vi "BLM_ManualControl.vi"() -> ()   [LabVIEW 2018]
doc: "To start rotations:\n\nSelect The Motor (BLM) address\nRun this VI\nClick Test connection button\nClick INITIALIZE button \n (It is assumed that a BLM controller should be initialized only once: immediately after it is turned on. \n E.g., usually there is no need to initialize if you rebooted computer, but kept the motor controller on,\n the motor was connected to the controller and you wish to continue using current position counting. \n Initialization occurs only if the current motor position is equal to zero.) \nClick READ BLM position button\nSelect desired MODE, SPEED, and Distance (or Final Position, depends on the MODE) value\nClick RUN BLM button\n\nSET POSITION button does not affect actual sample/motor position, but changes the position value\nin the controller memory. Thus, it allows to assign any value to the current motor position.\n\nSee also:\nhttps://opswiki.magnet.fsu.edu/wiki/pages/K7Q8u4C4s9/Rotating_probes_equipped_with_Brushless_Motors_BLMs.html\n\nNHMFL; A.Suslov; Feb 2012; updated Aug 2016"
uses:
  IMS Stepper Controller/stepper motor action.ctl
  slider setter action.ctl
panel:
  out "Error Out":errorcluster {"code" format="%.0x"}
  in  "MODE:":enum32{"ABSOLUTE", "INCREMENTAL"}(radio)=enum."INCREMENTAL"
  in  "Read Position":bool
  out "Test Results":string
  in  "Test Connection":bool
  out "BLM Position":dbl caption="BLM position\nincrement 0.045 \n (deg of BLM)" format="%.3f"
  in  "Parameter changed":bool
  in  "stop":bool
  in  "Set Position":bool
  in  "INITIALIZE":bool
  in  "Run":bool
  in  "New position":dbl caption="Final position:\nincrement 0.045 \n (deg of BLM)" step=0.045 format="%#.3g"
  in  "SPEED (rot/sec)\nincrement .0042":dbl=0.0294 min=0.0042 max=0.42 step=0.0042
  in  "MOTOR (BLM) Address":refnum<visa-resource-name>
  # "Select The Motor (BLM) address\nRun this VI\nClick Test connection button\nClick  INITIALIZE button \nClick  READ BLM position button\nSelect desired MODE, SPEED, and\n         Distance (or Final Position)\nClick RUN BLM button\n\nMore Help at File-> VI Propeties->\nDocumentation\nand Operations Wiki"
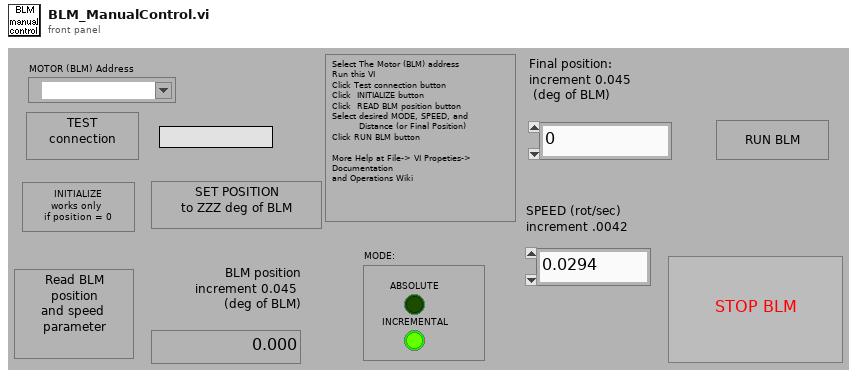
[diagram p1: front panel]
types:
  T1 = typedef "stepper motor action.ctl" = enum16{"go", "stop", "check", "init", "sync", "set", "set speed", "void"}
  T2 = enum8{"Enabled", "Disabled", "Disabled and Grayed Out"}
  T3 = typedef "slider setter action.ctl" = enum16{"--update circle", "set step slider moves", "cursor moves", "current pos changed", "init", "void", "--draw current lie", "--draw set line", "--move current step slider", "--move set step slider", "--draw limit lines", "check", "--move set angle slider", "--move current angle slider", "set angle slider moves", "--move cursor", "set set step", "set current step"}
  T4 = typedef "stepper motor state.ctl" = enum16{"moving", "stopped"}
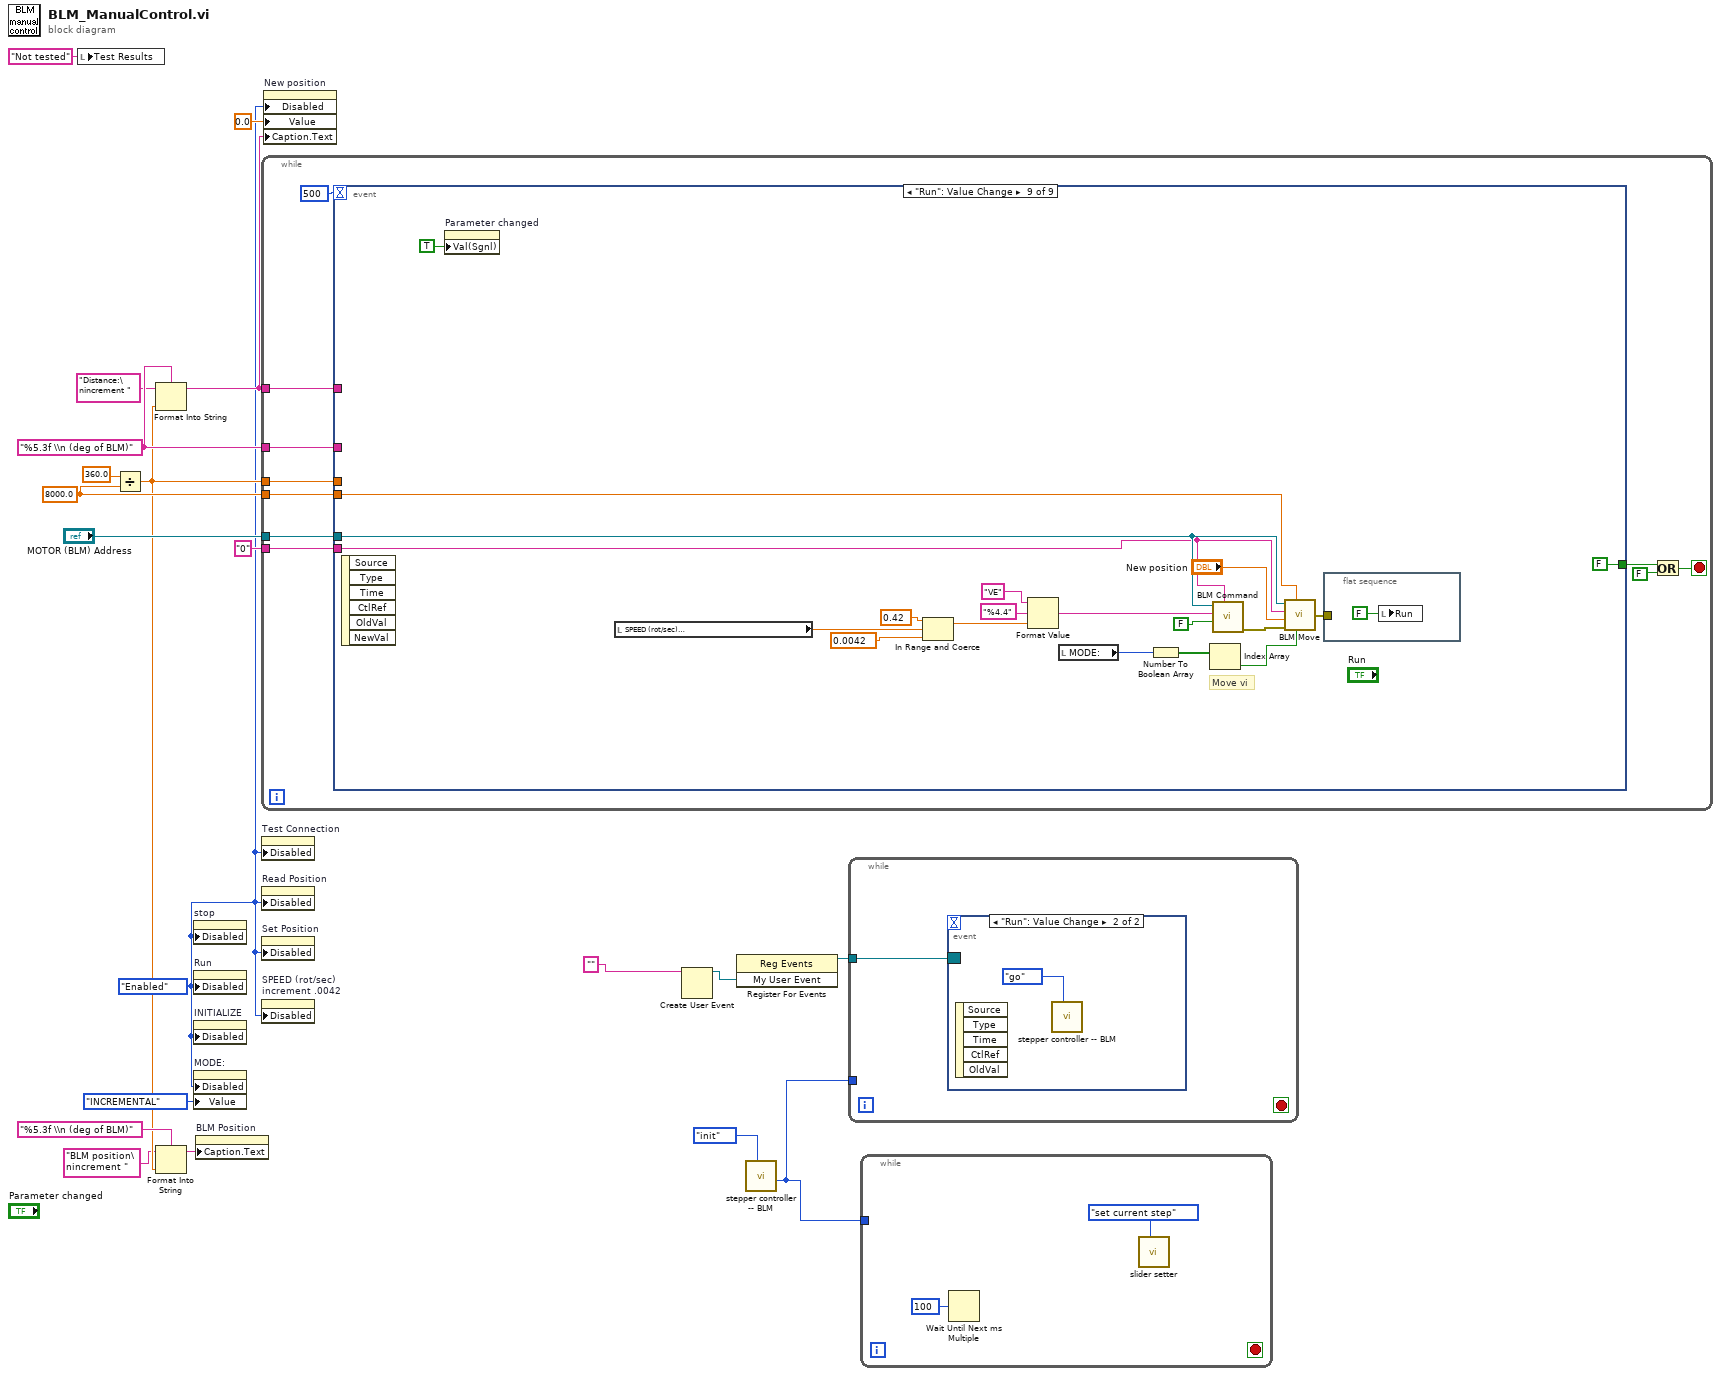
[diagram p0: block diagram]
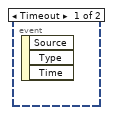
[diagram p2: hidden frame]
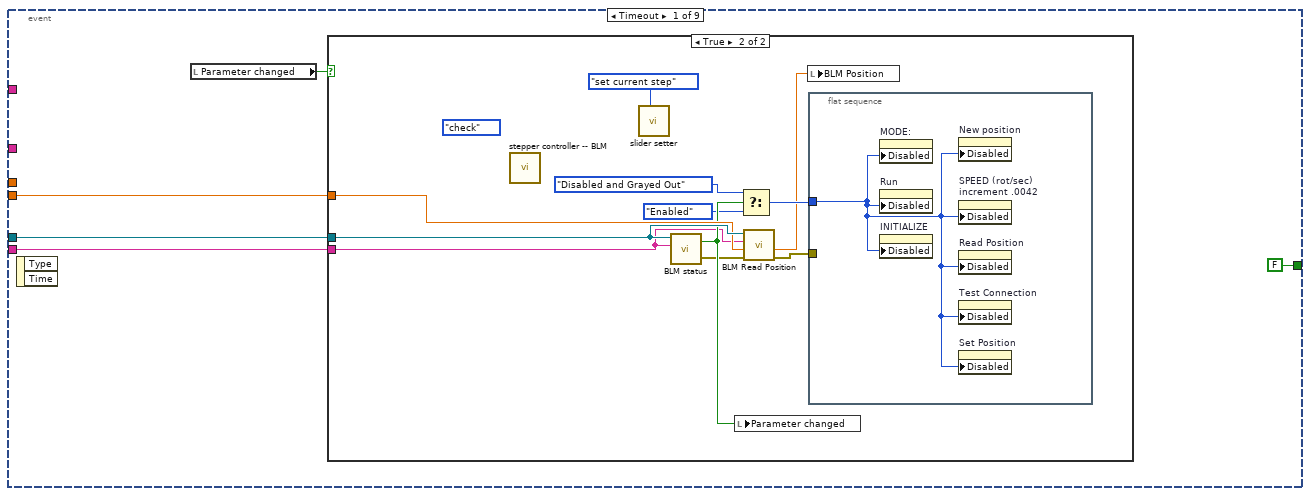
[diagram p3: hidden frame]
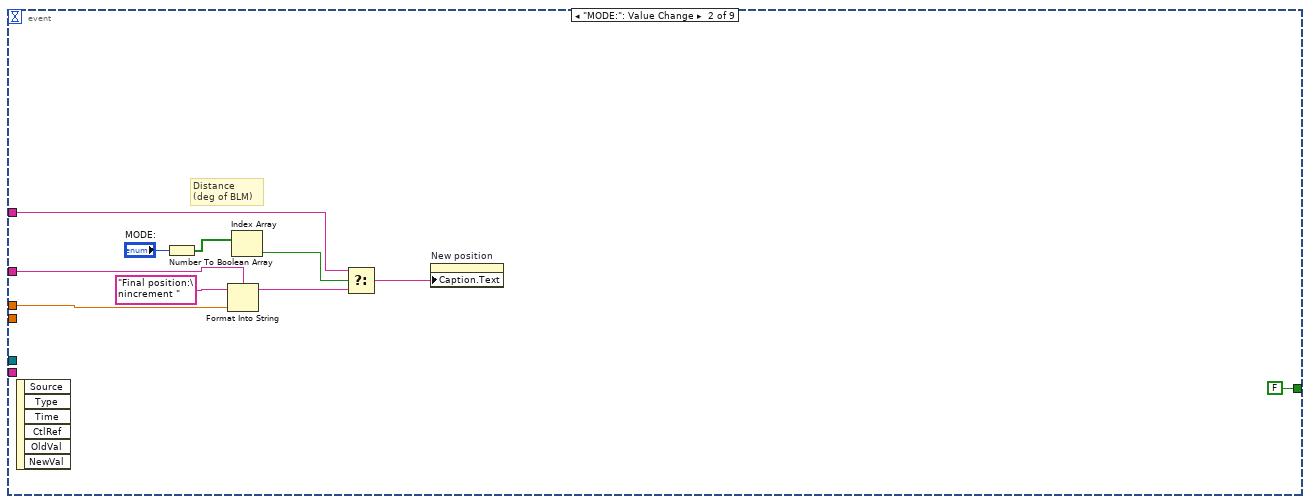
[diagram p5: hidden frame]
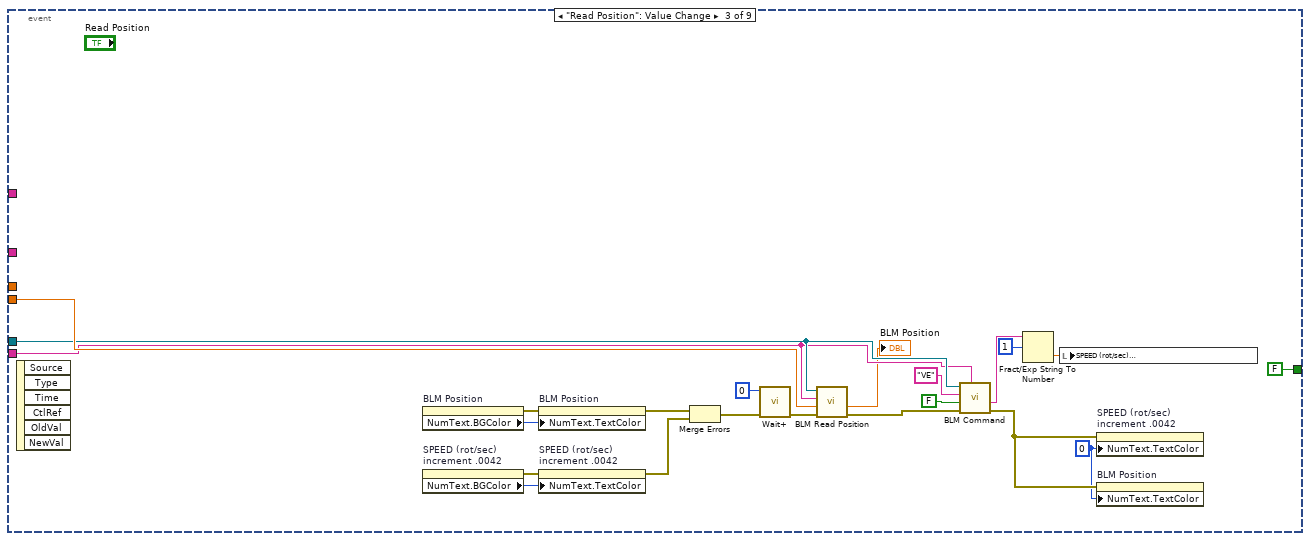
[diagram p6: hidden frame]
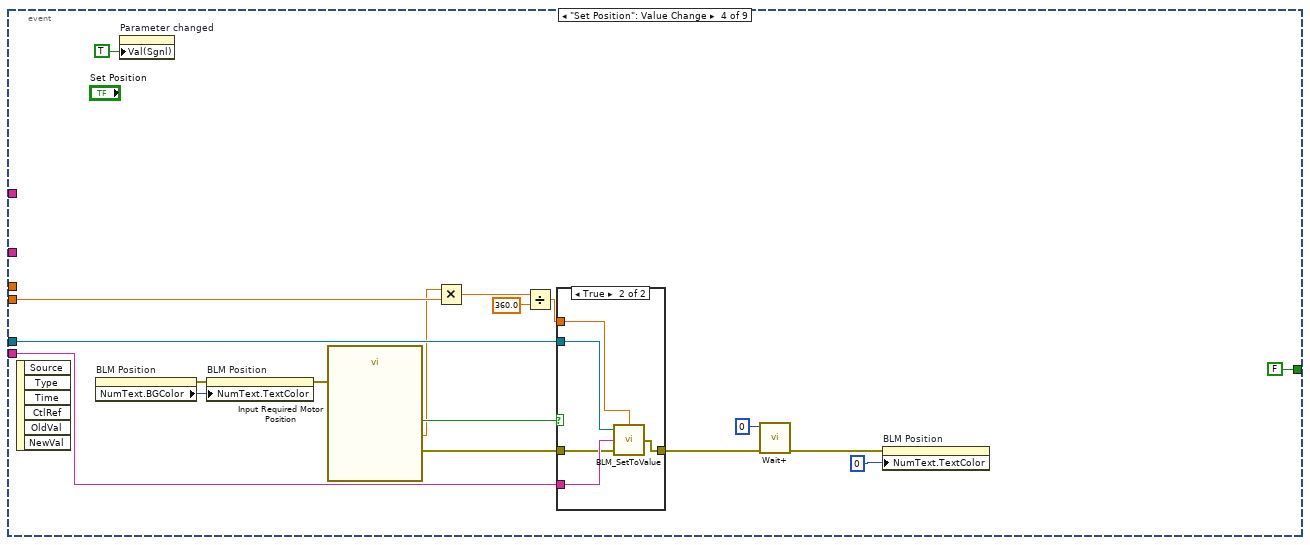
[diagram p7: hidden frame]
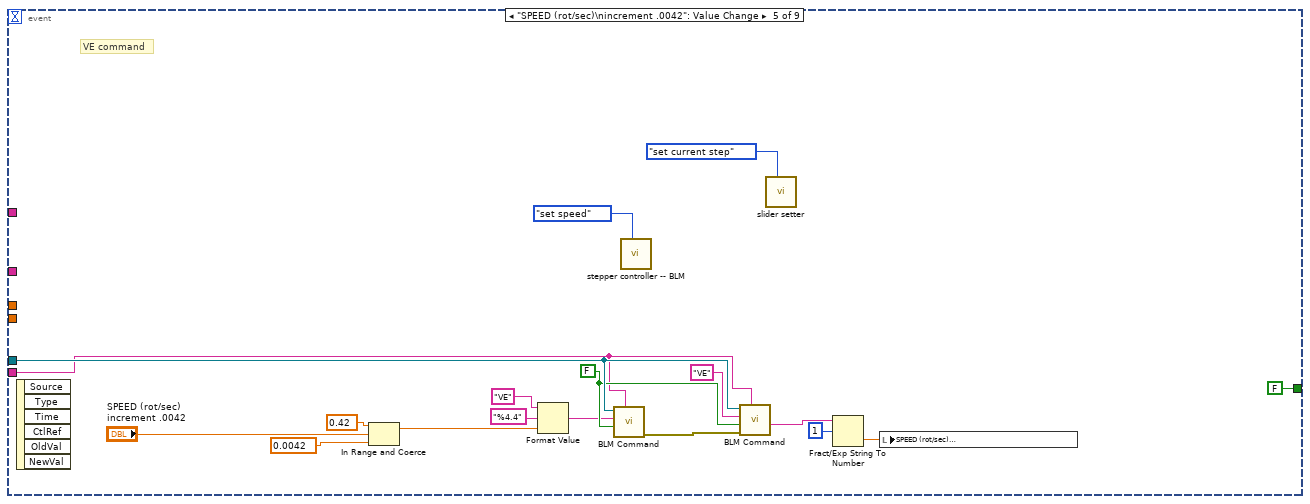
[diagram p9: hidden frame]
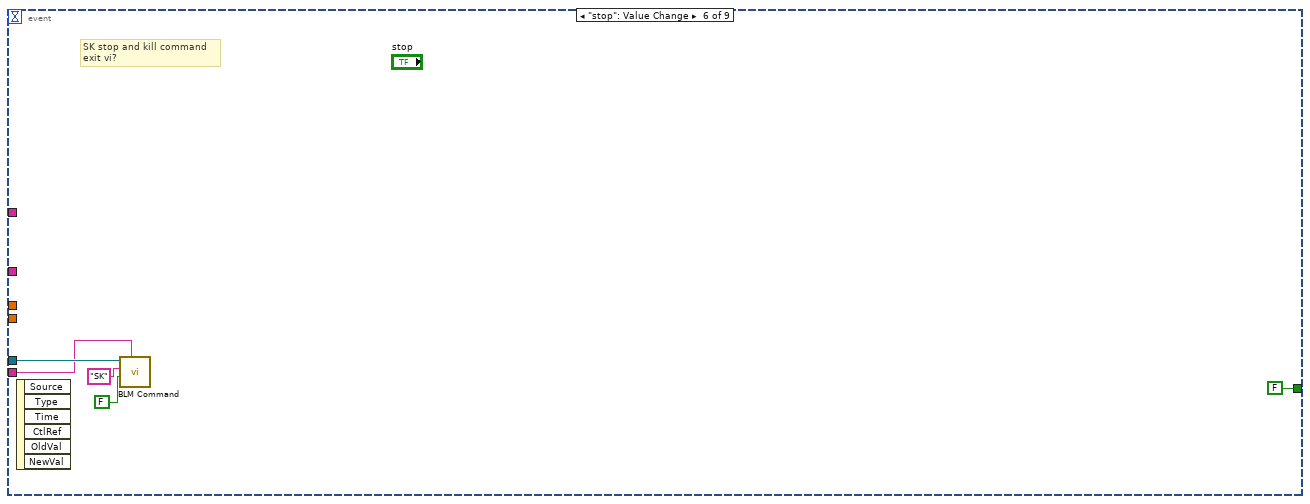
[diagram p10: hidden frame]
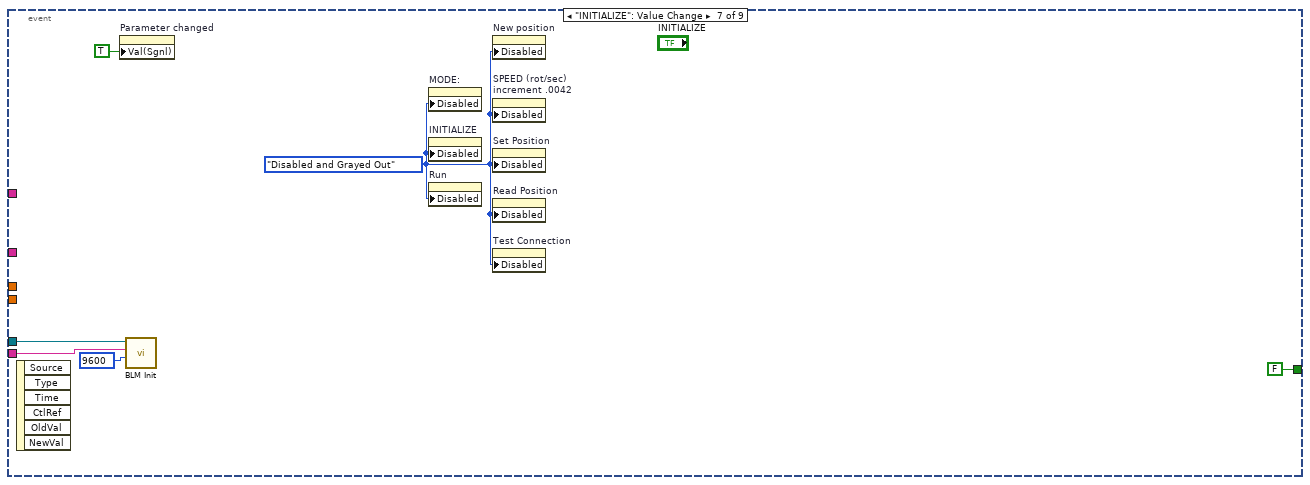
[diagram p11: hidden frame]
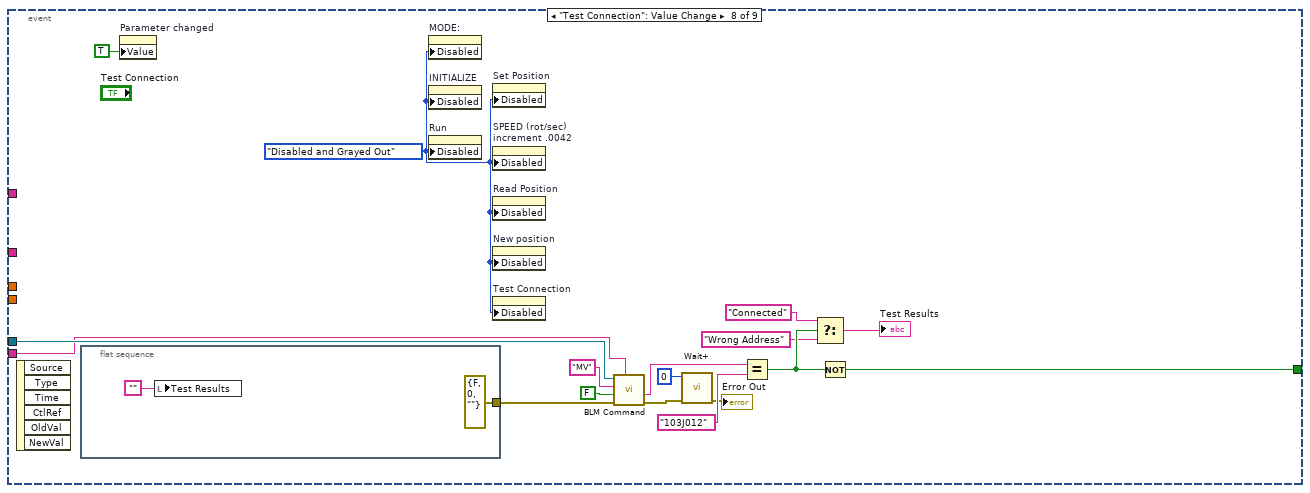
[diagram p12: hidden frame]
diagram:
  w7 = T2."Enabled" ("Disabled")
  w13 = "%5.3f \\n (deg of BLM)" ("format string")
  w15 = 8000.0 ("Steps/rot")
  n1 = local write "Test Results"("Not tested" ("s? t:f")) -> ()
  n2 = Divide(x=360.0, y=w15) -> (x/y=w10:dbl)
  n3 = Format Into String(format string=w13, initial string="Distance:\nincrement " ("Label.Text"), w10) -> (resulting string=w14:string)  [unwired: 1 in, 1 out]
  n4 = Format Into String(format string="%5.3f \\n (deg of BLM)", initial string="BLM position\nincrement ", w10) -> (resulting string=w11:string)  [unwired: 1 in, 1 out]
  n5 = property on="stop" class="Bool"("Disabled"=w7) -> ()  [unwired: 2 in, 2 out]
  n6 = property on="Run" class="Bool (strict)"("Disabled"=w7) -> ()  [unwired: 2 in, 2 out]
  n7 = property on="INITIALIZE" class="Bool"("Disabled"=w7) -> ()  [unwired: 2 in, 2 out]
  n8 = property on="MODE:" class="RadioBtnsControl (strict)"("Disabled"=w7, "Value"=enum32{"ABSOLUTE", "INCREMENTAL"}."INCREMENTAL" ("MODE:")) -> ()  [unwired: 2 in, 2 out]
  n9 = property on="BLM Position" class="DigNum (strict)"("Caption.Text"=w11) -> ()  [unwired: 2 in, 2 out]
  n10 = while {
    tunnel: w15 -> [w30]
    tunnel: "MOTOR (BLM) Address" -> [w29]
    tunnel: w14 -> [w24]
    tunnel: "0" ("Motor Address") -> [w23]
    tunnel: w10 -> [w22]
    tunnel: w13 -> [w21]
    stop <- w26 stop-if-true
    n11 = event shown="[8] \"Run\": Value Change" {
      selector: _ -> [_ _ _ _ _ _ _ _ _]
      dyn-events: _ -> [_ _ _ _ _ _ _ _ _]
      timeout: 500 -> [_ _ _ _ _ _ _ _ _]
      tunnel: w30 -> [w34 _ w79 w94 _ _ _ _ w170]
      tunnel: w29 -> [w35 _ w78 w97 w121 w126 w131 w149 w169]
      tunnel: [FALSE FALSE FALSE FALSE FALSE FALSE FALSE w147 FALSE] -> w25
      tunnel: w24 -> [_ w56 _ _ _ _ _ _ _]
      tunnel: w23 -> [w32 _ w77 w95 w117 w123 w129 w145 w167]
      tunnel: w22 -> [_ w50 _ _ _ _ _ _ _]
      tunnel: w21 -> [_ w49 _ _ _ _ _ _ _]
      event Timeout {
        n12 = event-data() -> ()  [unwired: 1 in, 2 out]
        n13 = local read "Parameter changed"() -> (w33:bool)
        n14 = case shown="True" w33 {
          tunnel: w35 -> [_ w46]
          tunnel: w34 -> [_ w45]
          tunnel: w32 -> [_ w41]
          frame False {
          }
          frame True {
            (unwired) stepper_motor_action."check" ("stepper motor action")
            n15 = call "stepper controller -- BLM.vi"() -> ()  [unwired: 11 in, 1 out]
            n16 = call "slider setter.vi"("slider setter action"=slider_setter_action."set current step") -> ()  [unwired: 10 in, 1 out]
            n17 = call "BLM status.vi"("Motor Address"=w41, "Porty Address"=w46) -> ("error out"=w40:errorcluster, "Motor is moving"=w44:bool)  [unwired: 2 in]
            n18 = local write "Parameter changed"(w44) -> ()
            n19 = Select(t=T2."Disabled and Grayed Out" ("Disabled"), s=w44, f=T2."Enabled" ("Disabled")) -> (s? t:f=w43:T2)
            n20 = call "BLM Read Position.vi"("error in (no error)"=w40, "Steps/rot"=w45, "Motor Address"=w41, "Port Address"=w46) -> ("error out"=w39:errorcluster, "Response"=w42:dbl)  [unwired: 2 out]
            n21 = local write "BLM Position"(w42) -> ()
            n22 = flat-sequence {
              tunnel: w43 -> [w47]
              tunnel: w39 -> [_]
              frame #0 {
                n23 = property on="MODE:" class="RadioBtnsControl (strict)"("Disabled"=w47) -> ()  [unwired: 2 in, 2 out]
                n24 = property on="Run" class="Bool (strict)"("Disabled"=w47) -> ()  [unwired: 2 in, 2 out]
                n25 = property on="INITIALIZE" class="Bool"("Disabled"=w47) -> ()  [unwired: 2 in, 2 out]
                n26 = property on="New position" class="DigNum (strict)"("Disabled"=w47) -> ()  [unwired: 2 in, 2 out]
                n27 = property on="SPEED (rot/sec)\nincrement .0042" class="DigNum (strict)"("Disabled"=w47) -> ()  [unwired: 2 in, 2 out]
                n28 = property on="Read Position" class="Bool"("Disabled"=w47) -> ()  [unwired: 2 in, 2 out]
                n29 = property on="Test Connection" class="Bool"("Disabled"=w47) -> ()  [unwired: 2 in, 2 out]
                n30 = property on="Set Position" class="Bool"("Disabled"=w47) -> ()  [unwired: 2 in, 2 out]
              }
            }
          }
        }
      }
      event "MODE:": Value Change {
        # "Distance  \n(deg of BLM)"
        n31 = event-data() -> ()  [unwired: 1 in, 6 out]
        n32 = Number To Boolean Array(number="MODE:") -> (Boolean array=w54:bool[])
        n33 = Format Into String(format string=w49, initial string="Final position:\nincrement " ("f"), w50) -> (resulting string=w52:string)  [unwired: 1 in, 1 out]
        n34 = Index Array(array=w54) -> (element=w53:bool)  [unwired: 1 in]
        n35 = Select(t=w56, s=w53, f=w52) -> (s? t:f=w57:string)
        n36 = property on="New position" class="DigNum (strict)"("Caption.Text"=w57) -> ()  [unwired: 2 in, 2 out]
      }
      event "Read Position": Value Change {
        w64 = u32 0 ("Numeric Text.Text Colors:Text Color")
        n37 = event-data() -> ()  [unwired: 1 in, 6 out]
        n38 = property on="BLM Position" class="DigNum (strict)"() -> (error out=w58:errorcluster, "NumText.BGColor"=w63:u32)  [unwired: 2 in, 1 out]
        n39 = property on="SPEED (rot/sec)\nincrement .0042" class="DigNum (strict)"() -> (error out=w59:errorcluster, "NumText.BGColor"=w62:u32)  [unwired: 2 in, 1 out]
        n40 = property on="BLM Position" class="DigNum (strict)"(error in=w58, "NumText.TextColor"=w63) -> (error out=w61:errorcluster)  [unwired: 1 in, 1 out]
        n41 = property on="SPEED (rot/sec)\nincrement .0042" class="DigNum (strict)"(error in=w59, "NumText.TextColor"=w62) -> (error out=w60:errorcluster)  [unwired: 1 in, 1 out]
        n42 = Merge Errors(w61, w60) -> (w65:errorcluster)
        n43 = call "Wait+.vi"("Error In"=w65, "milliseconds to wait"=u32 0 ("millisecond timer value")) -> ("Error Out"=w67:errorcluster)  [unwired: 4 in, 1 out]
        n44 = call "BLM Read Position.vi"("error in (no error)"=w67, "Steps/rot"=w79, "Motor Address"=w77, "Port Address"=w78) -> ("error out"=w69:errorcluster, "Response"=→"BLM Position":dbl)  [unwired: 2 out]
        n45 = call "BLM Command.vi"("Motor Address"=w77, "error in (no error)"=w69, "Read Echo?"=FALSE, "Command"="VE", "Port Address"=w78) -> ("error out"=w75:errorcluster, "Response"=w72:string)  [unwired: 1 in, 3 out]
        n46 = Fract/Exp String To Number(string=w72, offset=1) -> (number=w70:dbl)  [unwired: 2 in, 1 out]
        n47 = local write "SPEED (rot/sec)\nincrement .0042"(w70) -> ()
        n48 = property on="SPEED (rot/sec)\nincrement .0042" class="DigNum (strict)"(error in=w75, "NumText.TextColor"=w64) -> ()  [unwired: 1 in, 2 out]
        n49 = property on="BLM Position" class="DigNum (strict)"(error in=w75, "NumText.TextColor"=w64) -> ()  [unwired: 1 in, 2 out]
      }
      event "Set Position": Value Change {
        n50 = event-data() -> ()  [unwired: 1 in, 6 out]
        n51 = property on="BLM Position" class="DigNum (strict)"() -> (error out=w80:errorcluster, "NumText.BGColor"=w89:u32)  [unwired: 2 in, 1 out]
        n52 = property on="Parameter changed" class="Bool (strict)"("Val(Sgnl)"=TRUE ("Value (Signaling)")) -> ()  [unwired: 2 in, 2 out]
        n53 = property on="BLM Position" class="DigNum (strict)"(error in=w80, "NumText.TextColor"=w89) -> (error out=w90:errorcluster)  [unwired: 1 in, 1 out]
        n54 = call "Input Required Motor Position"("error in (no error)"=w90) -> ("Position:"=w87:dbl, "OK"=w88:bool, "error out"=w83:errorcluster)  [unwired: 16 in]
        n55 = Multiply(x=w87, y=w94) -> (x*y=w85:dbl)
        n56 = Divide(x=w85, y=360.0) -> (x/y=w86:dbl)
        n57 = case shown="True" w88 {
          tunnel: w97 -> [_ w103]
          tunnel: w95 -> [_ w102]
          tunnel: w86 -> [_ w101]
          tunnel: [w98 w100] -> w92
          tunnel: w83 -> [w98 w99]
          frame False {
          }
          frame True {
            n58 = call "BLM_SetToValue.vi"("Position"=w101, "error in (no error)"=w99, "Motor Address"=w102, "Port Address"=w103) -> ("error out"=w100:errorcluster)
          }
        }
        n59 = call "Wait+.vi"("Error In"=w92, "milliseconds to wait"=u32 0) -> ("Error Out"=w91:errorcluster)  [unwired: 4 in, 1 out]
        n60 = property on="BLM Position" class="DigNum (strict)"(error in=w91, "NumText.TextColor"=u32 0 ("Numeric Text.Text Colors:Text Color")) -> ()  [unwired: 1 in, 2 out]
      }
      event "SPEED (rot/sec)\nincrement .0042": Value Change {
        w120 = FALSE
        # "VE command"
        n61 = event-data() -> ()  [unwired: 1 in, 6 out]
        n62 = In Range and Coerce(upper limit=0.42 ("x"), x="SPEED (rot/sec)\nincrement .0042", lower limit=0.0042) -> (coerced(x)=w113:dbl)  [unwired: 1 out]
        n63 = Format Value(string ("")="VE", format string="%4.4", value (0)=w113) -> (output string=w110:string)
        n64 = call "BLM Command.vi"("Motor Address"=w117, "Read Echo?"=w120, "Command"=w110, "Port Address"=w121) -> ("error out"=w118:errorcluster)  [unwired: 2 in, 4 out]
        n65 = call "stepper controller -- BLM.vi"("stepper driver action"=stepper_motor_action."set speed" ("stepper motor action")) -> ()  [unwired: 10 in, 1 out]
        n66 = call "BLM Command.vi"("Motor Address"=w117, "error in (no error)"=w118, "Read Echo?"=w120, "Command"="VE", "Port Address"=w121) -> ("Response"=w107:string)  [unwired: 1 in, 4 out]
        n67 = call "slider setter.vi"("slider setter action"=slider_setter_action."set current step") -> ()  [unwired: 10 in, 1 out]
        n68 = Fract/Exp String To Number(string=w107, offset=1) -> (number=w119:dbl)  [unwired: 2 in, 1 out]
        n69 = local write "SPEED (rot/sec)\nincrement .0042"(w119) -> ()
      }
      event "stop": Value Change {
        # "SK stop and kill command\nexit vi?"
        n70 = event-data() -> ()  [unwired: 1 in, 6 out]
        n71 = call "BLM Command.vi"("Motor Address"=w123, "Read Echo?"=FALSE, "Command"="SK", "Port Address"=w126) -> ()  [unwired: 2 in, 5 out]
      }
      event "INITIALIZE": Value Change {
        w127 = T2."Disabled and Grayed Out" ("Disabled")
        n72 = event-data() -> ()  [unwired: 1 in, 6 out]
        n73 = property on="Parameter changed" class="Bool (strict)"("Val(Sgnl)"=TRUE ("Value (Signaling)")) -> ()  [unwired: 2 in, 2 out]
        n74 = call "BLM Init.vi"("Baud Rate"=u32 9600, "Motor Address"=w129, "Port Address"=w131) -> ()  [unwired: 1 in, 3 out]
        n75 = property on="MODE:" class="RadioBtnsControl (strict)"("Disabled"=w127) -> ()  [unwired: 2 in, 2 out]
        n76 = property on="INITIALIZE" class="Bool"("Disabled"=w127) -> ()  [unwired: 2 in, 2 out]
        n77 = property on="Run" class="Bool (strict)"("Disabled"=w127) -> ()  [unwired: 2 in, 2 out]
        n78 = property on="New position" class="DigNum (strict)"("Disabled"=w127) -> ()  [unwired: 2 in, 2 out]
        n79 = property on="SPEED (rot/sec)\nincrement .0042" class="DigNum (strict)"("Disabled"=w127) -> ()  [unwired: 2 in, 2 out]
        n80 = property on="Set Position" class="Bool"("Disabled"=w127) -> ()  [unwired: 2 in, 2 out]
        n81 = property on="Read Position" class="Bool"("Disabled"=w127) -> ()  [unwired: 2 in, 2 out]
        n82 = property on="Test Connection" class="Bool"("Disabled"=w127) -> ()  [unwired: 2 in, 2 out]
      }
      event "Test Connection": Value Change {
        w144 = T2."Disabled and Grayed Out" ("Disabled")
        n83 = event-data() -> ()  [unwired: 1 in, 6 out]
        n84 = flat-sequence {
          tunnel: [errorcluster {"status"=FALSE, "code"=0, "source"=""} ("error in (no error)")] -> w134
          frame #0 {
            n85 = local write "Test Results"("" ("Response")) -> ()
          }
        }
        n86 = property on="Parameter changed" class="Bool (strict)"("Value"=TRUE ("Parameter changed")) -> ()  [unwired: 2 in, 2 out]
        n87 = property on="MODE:" class="RadioBtnsControl (strict)"("Disabled"=w144) -> ()  [unwired: 2 in, 2 out]
        n88 = property on="INITIALIZE" class="Bool"("Disabled"=w144) -> ()  [unwired: 2 in, 2 out]
        n89 = property on="Run" class="Bool (strict)"("Disabled"=w144) -> ()  [unwired: 2 in, 2 out]
        n90 = property on="Set Position" class="Bool"("Disabled"=w144) -> ()  [unwired: 2 in, 2 out]
        n91 = property on="SPEED (rot/sec)\nincrement .0042" class="DigNum (strict)"("Disabled"=w144) -> ()  [unwired: 2 in, 2 out]
        n92 = property on="Read Position" class="Bool"("Disabled"=w144) -> ()  [unwired: 2 in, 2 out]
        n93 = property on="New position" class="DigNum (strict)"("Disabled"=w144) -> ()  [unwired: 2 in, 2 out]
        n94 = property on="Test Connection" class="Bool"("Disabled"=w144) -> ()  [unwired: 2 in, 2 out]
        n95 = call "BLM Command.vi"("Motor Address"=w145, "error in (no error)"=w134, "Read Echo?"=FALSE, "Command"="MV", "Port Address"=w149) -> ("error out"=w143:errorcluster, "Response"=w140:string)  [unwired: 1 in, 3 out]
        n96 = call "Wait+.vi"("Error In"=w143, "milliseconds to wait"=u32 0) -> ("Error Out"=→"Error Out":errorcluster)  [unwired: 4 in, 1 out]
        n97 = Equal?(x=w140, y="103J012" ("Response")) -> (x = y?=w148:bool)
        n98 = Select(t="Connected" ("Response"), s=w148, f="Wrong Address" ("Response")) -> (s? t:f=→"Test Results":string)
        n99 = Not(x=w148) -> (.not. x?=w147:bool)
      }
      event "Run": Value Change {
        # "Move vi"
        n100 = event-data() -> ()  [unwired: 1 in, 6 out]
        n101 = property on="Parameter changed" class="Bool (strict)"("Val(Sgnl)"=TRUE ("Value (Signaling)")) -> ()  [unwired: 2 in, 2 out]
        n102 = local read "SPEED (rot/sec)\nincrement .0042"() -> (w168:dbl)
        n103 = In Range and Coerce(upper limit=0.42 ("x"), x=w168, lower limit=0.0042) -> (coerced(x)=w162:dbl)  [unwired: 1 out]
        n104 = Format Value(string ("")="VE", format string="%4.4", value (0)=w162) -> (output string=w158:string)
        n105 = local read "MODE:"() -> (w154:enum32{"ABSOLUTE", "INCREMENTAL"})
        n106 = Number To Boolean Array(number=w154) -> (Boolean array=w155:bool[])
        n107 = Index Array(array=w155) -> (element=w153:bool)  [unwired: 1 in]
        n108 = call "BLM Command.vi"("Motor Address"=w167, "Read Echo?"=FALSE, "Command"=w158, "Port Address"=w169) -> ("error out"=w166:errorcluster)  [unwired: 2 in, 4 out]
        n109 = call "BLM Move.vi"("Mode IS:"=w153, "Steps/rot"=w170, "error in (no error)"=w166, "Position / Distance"="New position", "Motor Address"=w167, "Port Address"=w169) -> ("error out"=w165:errorcluster)
        n110 = flat-sequence {
          tunnel: w165 -> [_]
          frame #0 {
            n111 = local write "Run"(FALSE ("Run")) -> ()
          }
        }
      }
    }
    n112 = Or(x=w25, y=FALSE) -> (x .or. y?=w26:bool)
  }
  n113 = property on="Test Connection" class="Bool"("Disabled"=w7) -> ()  [unwired: 2 in, 2 out]
  n114 = property on="Read Position" class="Bool"("Disabled"=w7) -> ()  [unwired: 2 in, 2 out]
  n115 = property on="Set Position" class="Bool"("Disabled"=w7) -> ()  [unwired: 2 in, 2 out]
  n116 = property on="SPEED (rot/sec)\nincrement .0042" class="DigNum (strict)"("Disabled"=w7) -> ()  [unwired: 2 in, 2 out]
  n117 = property on="New position" class="DigNum (strict)"("Disabled"=w7, "Value"=0.0 ("New position / \n distance (deg of BLM)"), "Caption.Text"=w14) -> ()  [unwired: 2 in, 2 out]
  n118 = Create User Event(user event datatype="") -> (user event=w3:refnum<user-event>)  [unwired: 1 in, 1 out]
  n119 = register-events(w3) -> (reference out=w5:refnum<event-registration>)  [unwired: 2 in, 1 out]
  n120 = call "stepper controller -- BLM.vi"("stepper driver action"=stepper_motor_action."init" ("stepper motor action")) -> ("stepper motor state OUT"=w1:T4)  [unwired: 10 in]
  n121 = while {
    tunnel: w5 -> [w172]
    tunnel: w1 -> [_]
    stop <- _ stop-if-true
    n122 = event shown="[1] \"Run\": Value Change" {
      selector: w172 -> [_ _]
      dyn-events: _ -> [_ _]
      timeout: _ -> [_ _]
      event Timeout {
        n123 = event-data() -> ()  [unwired: 1 in, 3 out]
      }
      event "Run": Value Change {
        n124 = event-data() -> ()  [unwired: 1 in, 5 out]
        n125 = call "stepper controller -- BLM.vi"("stepper driver action"=stepper_motor_action."go" ("stepper motor action")) -> ()  [unwired: 10 in, 1 out]
      }
    }
  }
  n126 = while {
    tunnel: w1 -> [_]
    stop <- _ stop-if-true
    n127 = Wait Until Next ms Multiple(millisecond multiple=u32 100) -> ()  [unwired: 1 out]
    n128 = call "slider setter.vi"("slider setter action"=slider_setter_action."set current step") -> ()  [unwired: 10 in, 1 out]
  }
